vi "Update TCP IP nodes with Test Machine IP.vi"(7 "nodepaths":string[](array[string]), 8 "error in (no error)":errorcluster, 11 "SysDef path in":path) -> (0 "error out":errorcluster, 3 "SysDef path out":path)   [LabVIEW 2018]
doc: "This VI is used to update the Instrument Addon TCP IP with the Machine IP."
uses:
  NationalInstruments.VeriStand.SystemDefinitionAPI
  niveristand-custom-device-testing-tools/VeriStandTestUtilities/VeriStandTestUtilities.lvlib
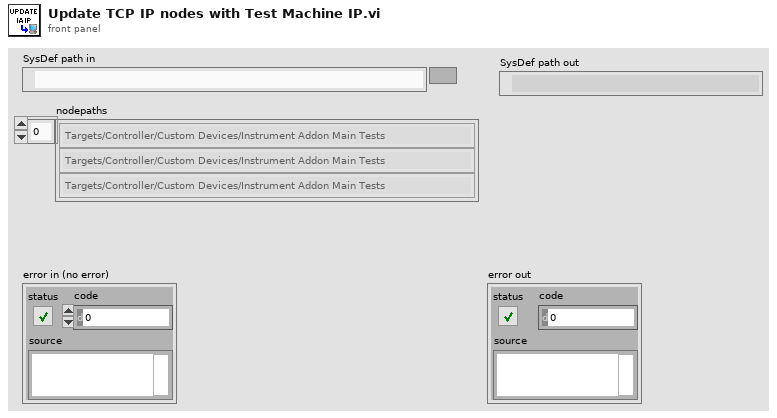
[diagram p1: front panel]
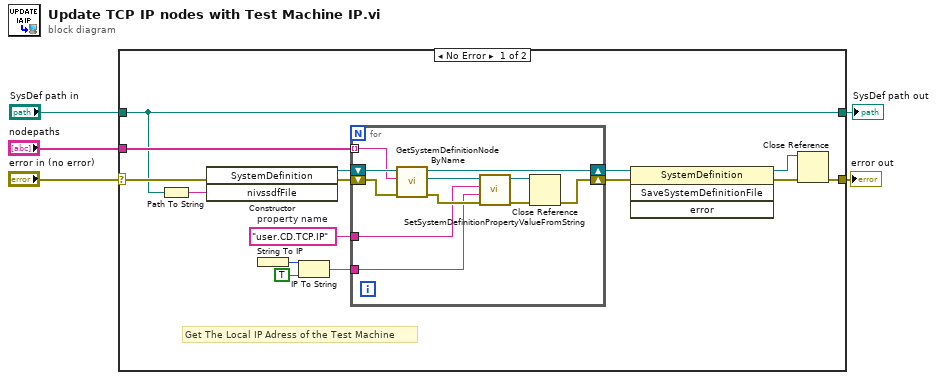
[diagram p0: block diagram]
diagram:
  n1 = case shown="No Error" "error in (no error)" {
    selector: "error in (no error)" -> [w7 w33]
    tunnel: "SysDef path in" -> [w6 w32]
    tunnel: "nodepaths" -> [w11 _]
    tunnel: [w8 w33] -> w3
    tunnel: [w6 w32] -> w1
    frame No Error {
      w13 = "user.CD.TCP.IP"  # property name
      # "Get The Local IP Adress of the Test Machine"
      n2 = Path To String(path=w6) -> (string=w18:string)
      n3 = constructor class="SystemDefinition"(error in=w7, "nivssdfFile"=w18) -> (reference out=w16:refnum<k24>, error out=w17:errorcluster)  [unwired: 2 in, 2 out]
      n4 = String To IP() -> (0:w20:u32)  [unwired: 1 in]
      n5 = IP To String(1:TRUE ("dot notation? (F)"), 2:w20) -> (0:w12:string)
      n6 = for {
        tunnel: w13 -> [w26]
        tunnel: w12 -> [w25]
        shift-right: [w21] -> w14
        shift-left: w17 -> [w30]
        shift-right: [w27] -> w15
        shift-left: w16 -> [w29]
        tunnel: w11 -> [w24] mode=indexing
        n7 = call "GetSystemDefinitionNodeByName.vi"("error in (no error)"=w30, "nodepath"=w24, "SystemDefinition in"=w29) -> ("error out"=w31:errorcluster, "BaseNodeType"=w28:refnum<k24>, "SystemDefinition out"=w27:refnum<k24>)  [unwired: 6 in]
        n8 = call "SetSystemDefinitionPropertyValueFromString.vi"("error in (no error)"=w31, "value"=w25, "property name"=w26, "BaseNodeType in"=w28) -> ("error out"=w22:errorcluster, "BaseNodeType out"=w23:refnum<k24>)  [unwired: 6 in]
        n9 = Close Reference(reference=w23, error in (no error)=w22) -> (error out=w21:errorcluster)
      }
      n10 = invoke class="SystemDefinition" method="SaveSystemDefinitionFile"(reference=w15, error in=w14) -> (reference out=w9:refnum<k24>, error out=w10:errorcluster)  [unwired: 2 in, 2 out]
      n11 = Close Reference(reference=w9, error in (no error)=w10) -> (error out=w8:errorcluster)
    }
    frame Error {
    }
  }
  "error out" <- w3
  "SysDef path out" <- w1
